vi "Teste_Read_Meteorologica.vi"() -> (0 "Erro":bool)   [LabVIEW 2018]
uses:
  Global_Telescopio.vi
  Shared_160.lvlib
panel:
  in  "Case Constant\n(See Context Help)":bool
  out "error out":errorcluster
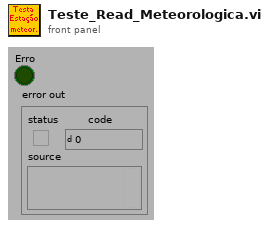
[diagram p1: front panel]
types:
  T1 = enum16{"open", "open or create", "create or replace", "create"}
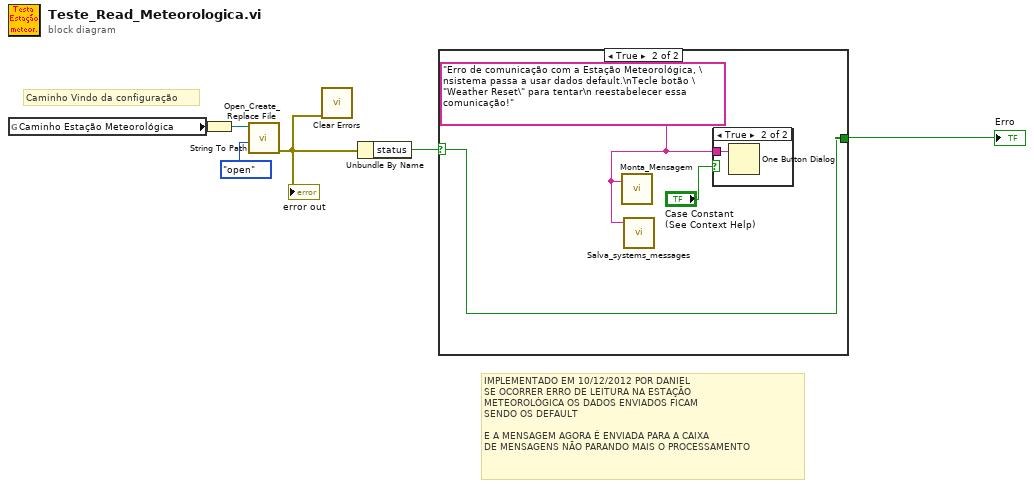
[diagram p0: block diagram]
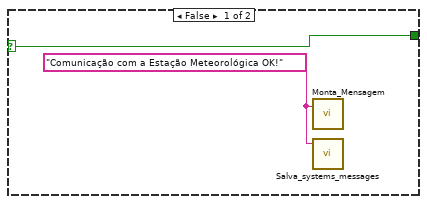
[diagram p2: hidden frame]
diagram:
  # "IMPLEMENTADO EM 10/12/2012 POR DANIEL\nSE OCORRER ERRO DE LEITURA NA ESTAÇÃO\nMETEOROLÓGICA OS DADOS ENVIADOS FICAM\nSENDO OS DEFAULT\n\nE A MENSAGEM AGORA É ENVIADA PARA A CAIXA\nDE MENSAGENS NÃO PARANDO MAIS O PROCESSAMENTO"
  # "Caminho Vindo da configuração"
  n1 = global read "Global_Telescopio.vi" "Caminho Estação Meteorológica"() -> (w4:string)
  n2 = String To Path(string=w4) -> (path=w5:path)
  n3 = call <vilib>:"Open_Create_Replace File.vi"("function (open:0)"=T1."open", "file path"=w5) -> ("error out"=w3:errorcluster)  [unwired: 6 in, 3 out]
  "error out" <- w3
  n4 = call <vilib>:"Clear Errors.vi"("error in (no error)"=w3) -> ()  [unwired: 5 in, 2 out]
  n5 = Unbundle By Name(w3) -> ("status"=w1:bool)
  n6 = case shown="True" w1 {
    selector: w1 -> [w8 w11]
    tunnel: [w8 w11] -> w2
    frame False {
      w7 = "Comunicação com a Estação Meteorológica OK!" ("message")
      n7 = call "Monta_Mensagem.vi"("Mensagem"=w7) -> ()  [unwired: 2 in]
      n8 = call "Salva_systems_messages.vi"("Mensagem"=w7) -> ()  [unwired: 5 in]
    }
    frame True {
      w9 = "Erro de comunicação com a Estação Meteorológica, \nsistema passa a usar dados default.\nTecle botão \"Weather Reset\" para tentar\n reestabelecer essa comunicação!" ("message")
      n9 = call "Monta_Mensagem.vi"("Mensagem"=w9) -> ()  [unwired: 2 in]
      n10 = call "Salva_systems_messages.vi"("Mensagem"=w9) -> ()  [unwired: 5 in]
      n11 = case shown="True" "Case Constant\n(See Context Help)" {
        tunnel: w9 -> [_ w12]
        frame False {
        }
        frame True {
          n12 = One Button Dialog(message=w12) -> ()  [unwired: 1 in, 1 out]
        }
      }
    }
  }
  "Erro" <- w2
